vi "SpectrometerTestGrams.vi"() -> ()   [LabVIEW 2010]
panel:
  in  "User name":string
  in  "Output Path name":path
  out "Spectrum of the first Spectrometer":cluster{"Y":dbl[], "Y":dbl[]}[](graph)
  in  "stop":bool
  in  "Enter the \nInetegration Time":i32
  in  "Start":bool=TRUE
  out "Number of Spectrometers":i32
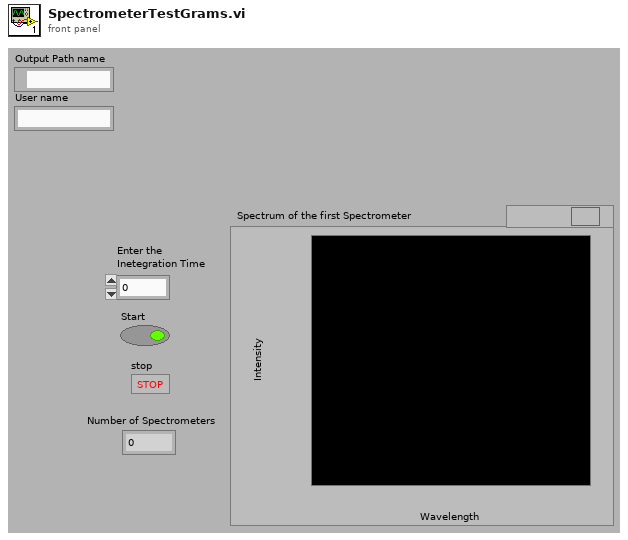
[diagram p1: front panel]
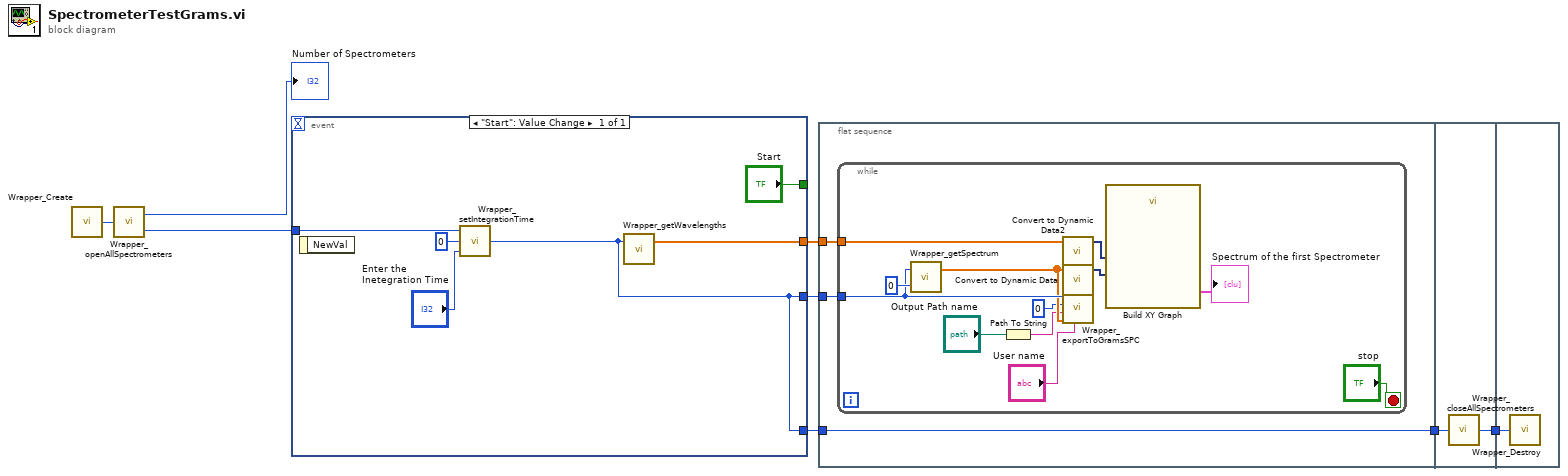
[diagram p0: block diagram]
diagram:
  n1 = call "Wrapper_Create.vi"() -> ("Wrapper"=w8:u32)
  n2 = call "Wrapper_openAllSpectrometers.vi"("Wrapper In"=w8) -> ("Number of Spectrometers"=→"Number of Spectrometers":i32, "Wrapper Out"=w6:u32)
  n3 = event shown="[0] \"Start\": Value Change" {
    selector: _ -> [_]
    dyn-events: _ -> [_]
    timeout: _ -> [_]
    tunnel: ["Start"] -> _
    tunnel: w6 -> [w11]
    tunnel: [w9] -> w5
    tunnel: [w10] -> w4
    tunnel: [w9] -> w2
    event "Start": Value Change {
      n4 = event-data() -> ()  [unwired: 2 out]
      n5 = call "Wrapper_setIntegrationTime.vi"("Integration Time"="Enter the \nInetegration Time", "Index"=0, "Wrapper In"=w11) -> ("Wrapper Out"=w9:u32)
      n6 = call "Wrapper_getWavelengths.vi"("Wrapper"=w9) -> ("WL Values"=w10:dbl[])  [unwired: 1 in, 1 out]
    }
  }
  n7 = flat-sequence {
    tunnel: w5 -> [w17]
    tunnel: w4 -> [w16]
    tunnel: [w15] -> w3
    tunnel: w2 -> [w15]
    tunnel: w3 -> [w31]
    tunnel: [w30] -> w1
    tunnel: w1 -> [w32]
    frame #0 {
      n8 = while {
        tunnel: w17 -> [w23]
        tunnel: w16 -> [w25]
        stop <- "stop" stop-if-true
        n9 = call "Wrapper_getSpectrum.vi"("Index"=0, "Wrapper"=w23) -> ("Spectrum Values"=w22:dbl[])  [unwired: 1 out]
        n10 = Path To String(path="Output Path name") -> (string=w18:string)
        n11 = call "Convert to Dynamic Data2"("Array"=w25) -> ("Dynamic Data Type"=w24:dynamicdata)  [unwired: 3 out]
        n12 = call "Convert to Dynamic Data"("Array"=w22) -> ("Dynamic Data Type"=w26:dynamicdata)  [unwired: 3 out]
        n13 = call "Wrapper_exportToGramsSPC.vi"("User name"="User name", "double_array"=w22, "Output Path name"=w18, "Index"=0, "Wrapper"=w23) -> ()  [unwired: 7 out]
        n14 = call "Build XY Graph"("Y Input"=w26, "X Input"=w24) -> ("XY Graph"=→"Spectrum of the first Spectrometer":cluster{"Y":dbl[], "Y":dbl[]}[])  [unwired: 3 in, 6 out]
      }
    }
    frame #1 {
      n15 = call "Wrapper_closeAllSpectrometers.vi"("Wrapper In"=w31) -> ("Wrapper Out"=w30:u32)
    }
    frame #2 {
      n16 = call "Wrapper_Destroy.vi"("Wrapper"=w32) -> ()
    }
  }
